vi "TestEventTransport_ValueOK.vi"(8 "error in (no error)":errorcluster, 11 "TestCase in":refnum<class "TestTransport.lvclass">) -> (0 "error out":errorcluster, 3 "TestCase out":refnum<class "TestTransport.lvclass">)   [LabVIEW 2015, in "Transport.lvlib" / "TestTransport.lvclass"]
uses:
  TestTransport.lvclass
  EventTransport/EventTransport.lvclass
panel:
  out "element":T1
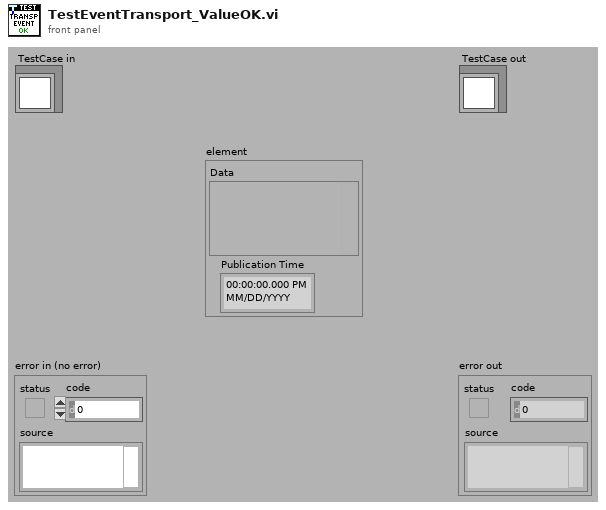
[diagram p1: front panel]
types:
  T1 = cluster{"Data":variant, "Publication Time":timestamp}
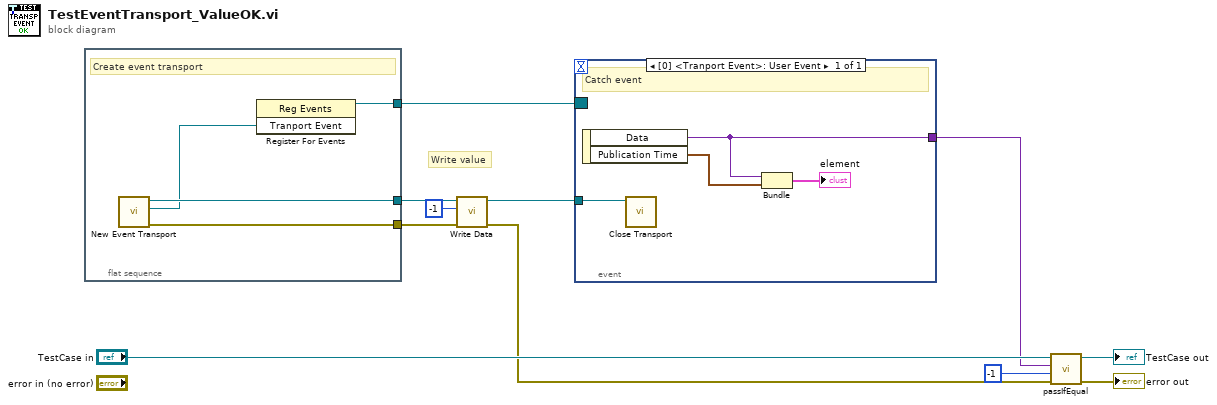
[diagram p0: block diagram]
diagram:
  # "Write value"
  n1 = flat-sequence {
    tunnel: [w15] -> w6
    tunnel: [w14] -> w5
    tunnel: [w12] -> w3
    frame #0 {
      # "Create event transport"
      n2 = call "New Event Transport.vi"() -> ("error out"=w14:errorcluster, "Tranport Event"=w13:refnum<user-event>, "EventTransport"=w15:refnum<class "EventTransport.lvclass">)  [unwired: 9 in]
      n3 = register-events(w13) -> (reference out=w12:refnum<event-registration>)  [unwired: 2 in, 1 out]
    }
  }
  n4 = call-dynamic "Write Data.vi"("error in (no error)"=w5, "Value"=-1, "EventTransport In"=w6) -> ("error out"=w2:errorcluster, "EventTransport Out"=w1:refnum<class "EventTransport.lvclass">)  [unwired: 7 in]
  n5 = event shown="[0] <Tranport Event>: User Event" {
    selector: w3 -> [_]
    dyn-events: _ -> [_]
    timeout: _ -> [_]
    tunnel: [w19] -> w4
    tunnel: w1 -> [w16]
    event User Event {
      # "Catch event"
      n6 = event-data() -> ("Data"=w19:variant, "Publication Time"=w18:timestamp)  [unwired: 1 in]
      n7 = call-dynamic "Close Transport.vi"("EventTransport in"=w16) -> ()  [unwired: 10 in, 1 out]
      n8 = Bundle("Data"=w19, "Publication Time"=w18) -> (→"element":T1)  [unwired: 1 in]
    }
  }
  n9 = call-dynamic "passIfEqual.vi"("error in (no error)"=w2, "y"=-1, "x"=w4, "TestCase in"="TestCase in") -> ("error out"=→"error out":errorcluster, "TestCase out"=→"TestCase out":refnum<class "TestTransport.lvclass">)  [unwired: 6 in]
